vi "Configure.vi"(0 "reference in":refnum<class "WebFrontPanel.lvclass">, 5 "error in (no error)":errorcluster) -> (14 "reference out":refnum<class "WebFrontPanel.lvclass">, 19 "error out":errorcluster)   [LabVIEW 2014, in "FrontPanelPublisher.lvlib" / "WebFrontPanel.lvclass"]
doc: "Configure the options for the web-representation of the front panel"
uses:
  WebFrontPanel.lvclass
  Controls/FPObjectConfiguration.ctl
  Control_class/Control.lvclass
  <vilib>/Utility/error.llb/DialogType.ctl
  Object_class/Object.lvclass
panel:
  in  "Exit":bool
  in  "Save":bool
  in  "Tab Control":enum32{"Controls", "Indicators"}(tab)
  in  "Controls":T1[](array[typedef])
  in  "Indicators":T1[](array[typedef])
  # "The following objects can be configured for the web front panel."
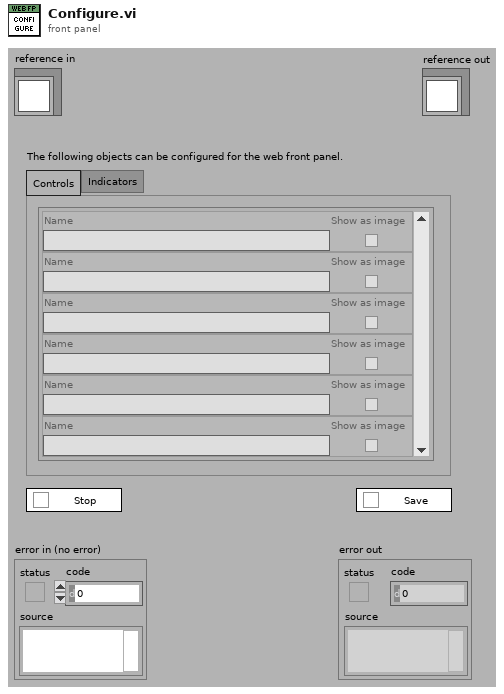
[diagram p1: front panel]
types:
  T1 = typedef "FrontPanelPublisher.lvlib/WebFrontPanel.lvclass/FPObjectConfiguration.ctl" = cluster{"Name":string, "Show as image":bool}
  T2 = enum32{"Invalid", "Standard", "Closed", "Hidden", "Minimized", "Maximized"}
  T3 = typedef "FrontPanelPublisher.lvlib/WebFrontPanel.lvclass/ObjectAttributes.ctl" = cluster{"VI Name":string, "VI Reference":refnum<vi>, "Controls":refnum<class "Object.lvclass">[], "Indicators":refnum<class "Object.lvclass">[], "Decorations":refnum<class "Object.lvclass">[]}
  T4 = typedef "DialogType.ctl" = u16
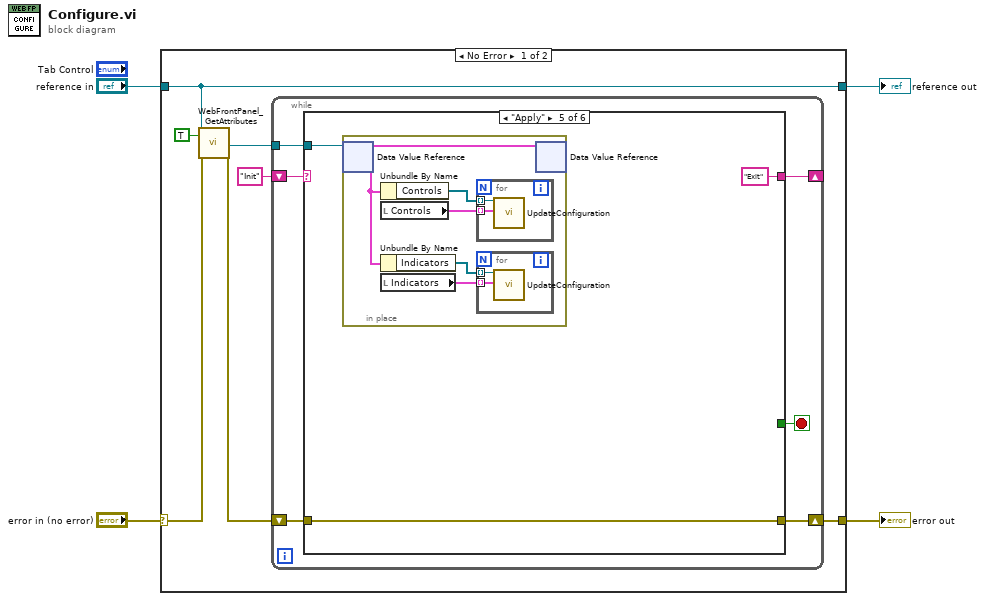
[diagram p0: block diagram]
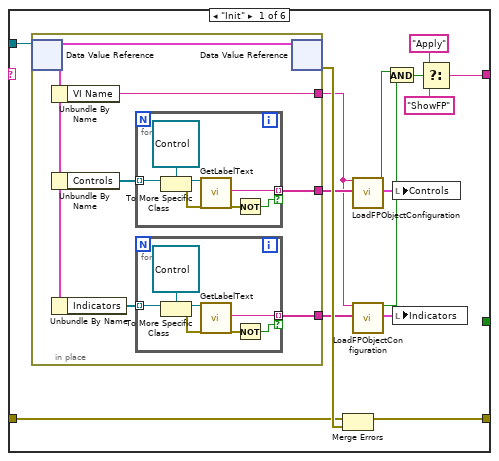
[diagram p2: hidden frame]
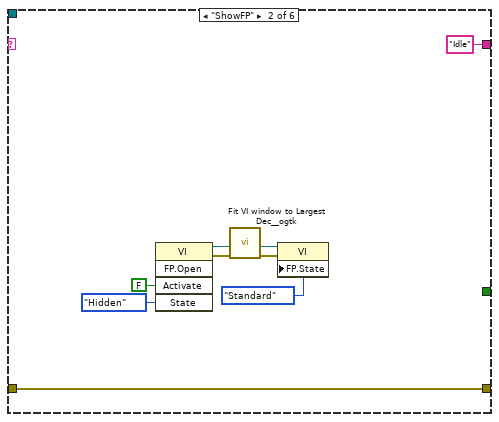
[diagram p3: hidden frame]
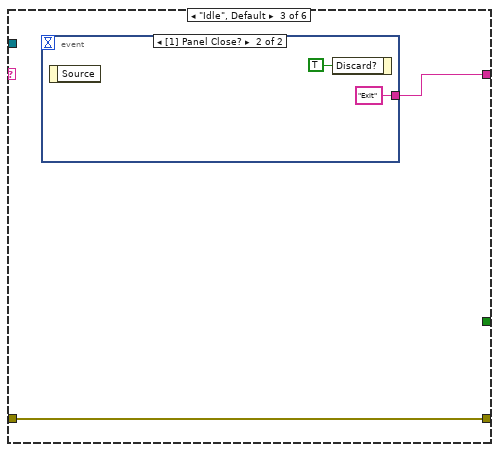
[diagram p4: hidden frame]
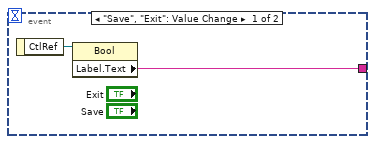
[diagram p5: hidden frame]
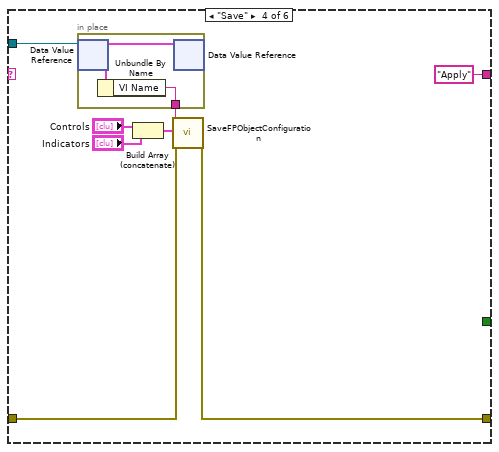
[diagram p6: hidden frame]
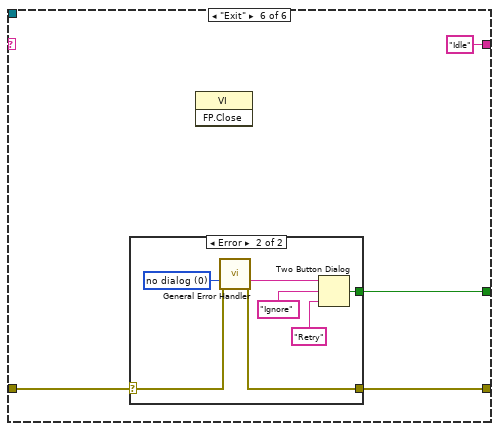
[diagram p7: hidden frame]
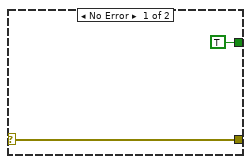
[diagram p8: hidden frame]
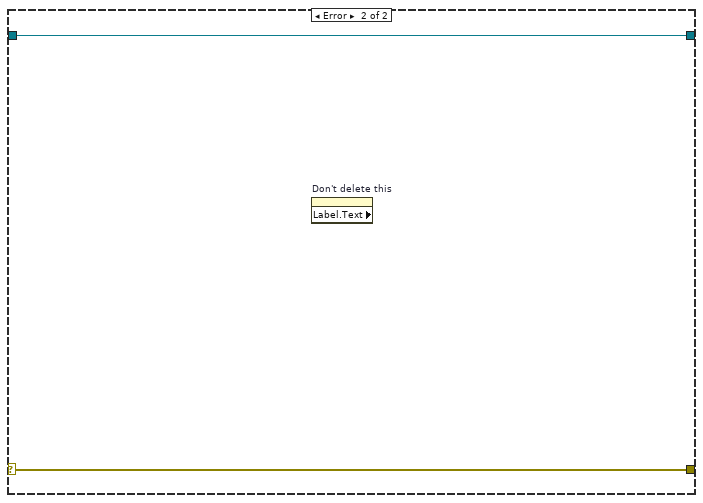
[diagram p9: hidden frame]
diagram:
  n1 = case shown="No Error" "error in (no error)" {
    selector: "error in (no error)" -> [w7 w103]
    tunnel: [w11 w103] -> w3
    tunnel: [w9 w102] -> w1
    tunnel: "reference in" -> [w9 w102]
    frame No Error {
      n2 = call "WebFrontPanel_GetAttributes.vi"("reference in"=w9, "OnlyGetDvrReference(False)"=TRUE, "error in (no error)"=w7) -> ("DataRef"=w8:refnum<data-value>, "error out"=w6:errorcluster)  [unwired: 13 in, 2 out]
      n3 = while {
        shift-right: [w16] -> w11
        shift-left: w6 -> [w17]
        shift-right: [w14] -> _
        shift-left: "Init" -> [w15]
        tunnel: w8 -> [w13]
        stop <- w12 stop-if-true
        n4 = case shown="\"Apply\"" w15 {
          tunnel: w17 -> [w24 w60 w61 w71 w77 w91]
          tunnel: [w31 w60 w61 w70 w77 w90] -> w16
          tunnel: [w19 "Idle" w62 "Apply" ("Label.Text") "Exit" ("Label.Text") "Idle" ("Label.Text")] -> w14
          tunnel: w13 -> [w25 _ _ w73 w79 _]
          tunnel: [_ _ _ _ _ w89] -> w12
          frame "Init" {
            n5 = in-place {
              in-place-border: [w36] -> w30
              in-place-border: [w34] -> w28
              in-place-border: [w33] -> w29
              n6 = in-place-dvr #1(w25) -> (w35:T3)  [unwired: 1 out]
              n7 = Unbundle By Name(w35) -> ("VI Name"=w34:string)
              n8 = Unbundle By Name(w35) -> ("Controls"=w38:refnum<class "Object.lvclass">[])
              n9 = Unbundle By Name(w35) -> ("Indicators"=w37:refnum<class "Object.lvclass">[])
              n10 = for {
                tunnel: w38 -> [w52] mode=indexing
                tunnel: [w48] -> w36 mode=indexing if=w46
                n11 = To More Specific Class(target class=refnum<class "Control.lvclass"> refnum ("FrontPanelPublisher.lvlib:Control"), reference=w52) -> (specific class reference=w51:refnum<class "Control.lvclass">, error out=w49:errorcluster)  [unwired: 1 in]
                n12 = call-dynamic "GetLabelText.vi"("reference in"=w51, "error in (no error)"=w49) -> ("Text"=w48:string, "error out"=w47:errorcluster)  [unwired: 15 in, 1 out]
                n13 = Not(x=w47) -> (.not. x?=w46:bool)
              }
              n14 = for {
                tunnel: w37 -> [w45] mode=indexing
                tunnel: [w41] -> w33 mode=indexing if=w39
                n15 = To More Specific Class(target class=refnum<class "Control.lvclass"> refnum ("FrontPanelPublisher.lvlib:Control"), reference=w45) -> (specific class reference=w44:refnum<class "Control.lvclass">, error out=w42:errorcluster)  [unwired: 1 in]
                n16 = call-dynamic "GetLabelText.vi"("reference in"=w44, "error in (no error)"=w42) -> ("Text"=w41:string, "error out"=w40:errorcluster)  [unwired: 15 in, 1 out]
                n17 = Not(x=w40) -> (.not. x?=w39:bool)
              }
              n18 = in-place-dvr #1(w35) -> (w32:errorcluster)  [unwired: 1 out]
            }
            n19 = Merge Errors(w24, w32) -> (w31:errorcluster)
            n20 = call "LoadFPObjectConfiguration.vi"("FP Name"=w28, "Objects"=w30) -> ("All Objects Configured"=w22:bool, "Objects Configurations"=w27:T1[])  [unwired: 16 in]
            n21 = call "LoadFPObjectConfiguration.vi"("FP Name"=w28, "Objects"=w29) -> ("All Objects Configured"=w23:bool, "Objects Configurations"=w26:T1[])  [unwired: 16 in]
            n22 = And(x=w22, y=w23) -> (x .and. y?=w21:bool)
            n23 = local write "Controls"(w27) -> ()
            n24 = local write "Indicators"(w26) -> ()
            n25 = Select(t="Apply", s=w21, f="ShowFP") -> (s? t:f=w19:string)
          }
          frame "ShowFP" {
            n26 = invoke class="VI" method="FP.Open"("Activate"=FALSE ("Activate?"), "State"=T2."Hidden") -> (reference out=w55:refnum<vi>, error out=w56:errorcluster)  [unwired: 3 in, 3 out]
            n27 = call <userlib>:"Fit VI window to Largest Dec__ogtk.vi"("error in (no error)"=w56) -> ("error out"=w53:errorcluster)  [unwired: 5 in, 1 out]
            n28 = property class="VI"(reference=w55, error in=w53, "FP.State"=T2."Standard" ("Front Panel Window:State")) -> ()  [unwired: 2 out]
          }
          frame "Idle", Default {
            n29 = event shown="[1] Panel Close?" {
              selector: _ -> [_ _]
              dyn-events: _ -> [_ _]
              timeout: _ -> [_ _]
              tunnel: [w63 "Exit" ("Label.Text")] -> w62
              event "Save", "Exit": Value Change {
                n30 = event-data() -> ("CtlRef"=w64:refnum<vi>)  [unwired: 1 in]
                n31 = property class="Bool"(reference=w64) -> ("Label.Text"=w63:string)  [unwired: 1 in, 2 out]
              }
              event Panel Close? {
                n32 = event-data() -> ()  [unwired: 1 in, 1 out]
                n33 = event-data("Discard?"=TRUE) -> ()  [unwired: 1 in, 1 out]
              }
            }
          }
          frame "Save" {
            n34 = in-place {
              in-place-border: [w76] -> w72
              n35 = in-place-dvr #2(w73) -> (w75:T3)  [unwired: 1 out]
              n36 = Unbundle By Name(w75) -> ("VI Name"=w76:string)
              n37 = in-place-dvr #2(w75) -> ()  [unwired: 2 out]
            }
            n38 = Build Array (concatenate)("Controls", "Indicators") -> (w74:T1[])
            n39 = call "SaveFPObjectConfiguration.vi"("FP Name"=w72, "Objects Configurations"=w74, "error in (no error)"=w71) -> ("error out"=w70:errorcluster)  [unwired: 16 in]
          }
          frame "Apply" {
            n40 = in-place {
              n41 = in-place-dvr #3(w79) -> (w84:T3)  [unwired: 1 out]
              n42 = Unbundle By Name(w84) -> ("Controls"=w83:refnum<class "Object.lvclass">[])
              n43 = local read "Controls"() -> (w82:T1[])
              n44 = Unbundle By Name(w84) -> ("Indicators"=w81:refnum<class "Object.lvclass">[])
              n45 = local read "Indicators"() -> (w80:T1[])
              n46 = for {
                tunnel: w83 -> [w88] mode=indexing
                tunnel: w82 -> [w87] mode=indexing
                n47 = call-dynamic "UpdateConfiguration.vi"("reference in"=w88, "FP Configuration"=w87) -> ()  [unwired: 16 in, 2 out]
              }
              n48 = for {
                tunnel: w81 -> [w86] mode=indexing
                tunnel: w80 -> [w85] mode=indexing
                n49 = call-dynamic "UpdateConfiguration.vi"("reference in"=w86, "FP Configuration"=w85) -> ()  [unwired: 16 in, 2 out]
              }
              n50 = in-place-dvr #3(w84) -> ()  [unwired: 2 out]
            }
          }
          frame "Exit" {
            n51 = case shown="Error" w91 {
              selector: w91 -> [w94 w101]
              tunnel: [w94 w100] -> w90
              tunnel: [TRUE ("T button?") w95] -> w89
              frame No Error {
              }
              frame Error {
                w99 = T4 0 items=["no dialog", "OK message", "continue or stop message", "OK message + warnings", "continue/stop + warnings"] ("type of dialog (OK msg:1)")
                n52 = call <vilib>:"General Error Handler.vi"("type of dialog (OK msg:1)"=w99, "error in (no error)"=w101) -> ("message"=w98:string, "error out"=w100:errorcluster)  [unwired: 9 in, 3 out]
                n53 = Two Button Dialog(message=w98, 1:"Retry", 2:"Ignore" ("String")) -> (T button?=w95:bool)
              }
            }
            n54 = invoke class="VI" method="FP.Close"() -> ()  [unwired: 3 in, 3 out]
          }
        }
      }
    }
    frame Error {
      n55 = property on="Don't delete this" class="LVClassControl (strict)" props=["Label", "Text"]() -> ()  [unwired: 2 in, 3 out]
    }
  }
  "error out" <- w3
  "reference out" <- w1
